vi "TLMB_LatestAPLPath.vi"(8 "Error In":errorcluster, 9 "APL Search String":T1(ring), 11 "Folder Path":path=path "\\\\itnas.appl.ge.com\\technology/Electronics/InProcess/Software/ci_builds/2015_VA_Washer") -> (0 "Error Out":errorcluster, 1 "Report text":string, 2 "Found ?":bool, 3 "File Path":path=path "\\\\itnas.appl.ge.com\\technology/Electronics/InProcess/Software/ci_builds/2015_VA_Washer/2015-03-06_03-42-38(Build-1952)/Binaries/2015VAWasher_Param_QA_Cycle_1_62_99_1.apl")   [LabVIEW 2016, in "TLMB.lvlib"]
doc: "This VI will search for the most recent version of software apls and return its path. You can search for various firware or xml apls.\n\nIf not found it will return an empty path, as well and boolean and report text."
uses:
  Projects/TLMB.lvlib
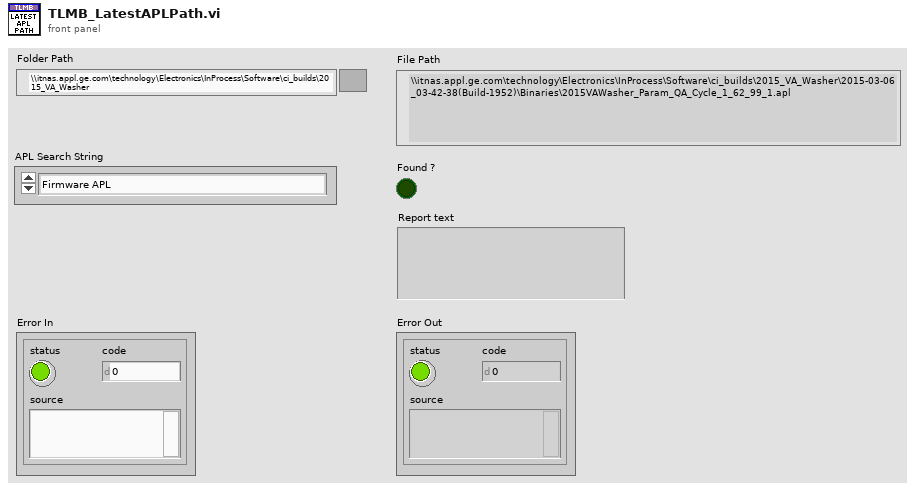
[diagram p1: front panel]
types:
  T1 = enum16{"Firmware APL", "System XML", "ERD Definitions XML"}
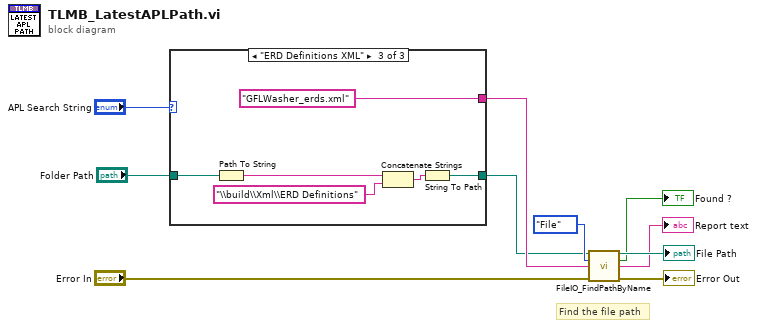
[diagram p0: block diagram]
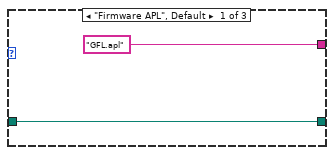
[diagram p2: hidden frame]
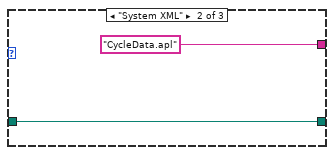
[diagram p3: hidden frame]
diagram:
  # "Find the file path"
  n1 = case shown="\"ERD Definitions XML\"" "APL Search String" {
    tunnel: ["GFL.apl" "CycleData.apl" "GFLWasher_erds.xml"] -> w7
    tunnel: [w11 w13 w15] -> w1
    tunnel: "Folder Path" -> [w11 w13 w16]
    frame "Firmware APL", Default {
    }
    frame "System XML" {
    }
    frame "ERD Definitions XML" {
      n2 = Path To String(path=w16) -> (string=w20:string)
      n3 = Concatenate Strings(w20, "\\build\\Xml\\ERD Definitions" ("string")) -> (w18:string)
      n4 = String To Path(string=w18) -> (path=w15:path)
    }
  }
  n5 = call "FileIO_FindPathByName.vi"("Path In"=w1, "File or Folder ?"=enum16{"Folder", "File"}."File", "File/Folder Search String"=w7, "Error In"="Error In") -> ("Path Out"=→"File Path":path, "Found ?"=→"Found ?":bool, "Report Text"=→"Report text":string, "Error Out"=→"Error Out":errorcluster)  [unwired: 8 in]
